vi "SET Message.vi"(8 "error in (no error)":errorcluster, 10 "Data":string, 11 "Parent_Class in":refnum<class "Message_Distributor_Class.lvclass">) -> (0 "error out":errorcluster, 3 "Parent_Class out":refnum<class "Message_Distributor_Class.lvclass">)   [LabVIEW 2023, in "Actor_Message_Distributor.lvlib" / "Message_Distributor_Class.lvclass"]
uses:
  Message_Distributor_Class.lvclass
  Usr Ev/Distributor - Ctrl - Enum - Events.ctl
  Message_Distributor_Class.lvclass/Message_Distributor_Class.ctl
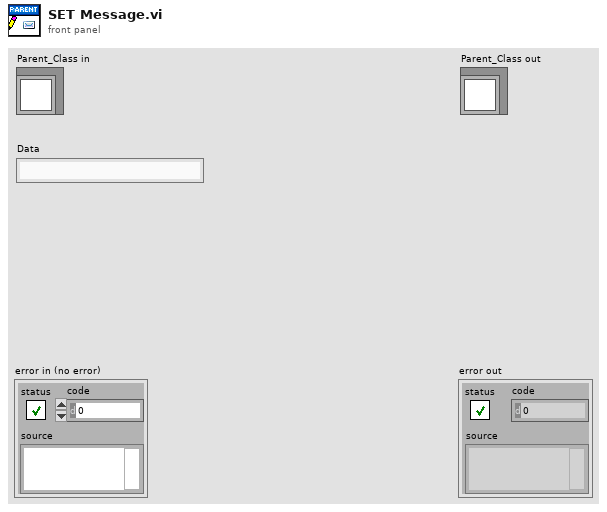
[diagram p1: front panel]
types:
  T1 = typedef "Actor_Message_Distributor.lvlib/Message_Distributor_Class.lvclass/Distributor - Ctrl - Enum - Events.ctl" = enum16{"SEND MESSAGE Ev", "STOP_ACTOR Ev", "INIT_ACTOR Ev", "START Ev", "STOP Ev", "GET Ev", "SET Ev", "ERROR_HANDLER Ev", "RESET Ev", "DISPATCH MESSAGE 2 CHILDS Ev", "ECU RESET Ev"}
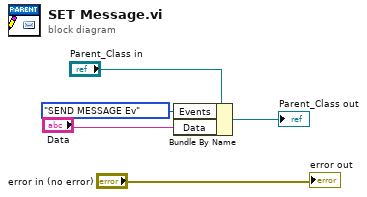
[diagram p0: block diagram]
diagram:
  n1 = Bundle By Name(cluster="Parent_Class in", "Events"=Distributor_-_Ctrl_-_Enum_-_Events."SEND MESSAGE Ev" ("Parent Trigger Event Cluster.Events"), "Data"="Data") -> (→"Parent_Class out":refnum<class "Message_Distributor_Class.lvclass">)
  "error out" <- "error in (no error)"
